vi "EncoderSpeedMise_original.vi"(8 "error in (no error)":errorcluster, 11 "Cluster in":T1={FALSE, "Tick Count(uSec)"=0, "Counter Value"=[0, 0, 0, 0], "x-y"=[0, 0, 0, 0]}) -> (0 "error out":errorcluster, 1 "Updated":bool, 2 "output cluster":T2, 3 "Cluster Out":T1, 4 "Tick Count(uSec)":u32 caption="Tick Count(Ticks)")   [LabVIEW 2018]
uses:
  <vilib>/myRIO/Common/Instrument Driver Framework/myRIO v1.0/Encoder/typedefs/Encoder Signal Mode.ctl
  <vilib>/myRIO/Instrument Drivers/Onboard IO/Encoder/typedefs/Encoder Reference.ctl
  <vilib>/myRIO/Common/Instrument Driver Framework/Utilities/typedefs/myRIO Generic Hardware Reference.ctl
  <vilib>/myRIO/Common/Instrument Driver Framework/Utilities/typedefs/Hardware Version Enum.ctl
  <vilib>/myRIO/Common/Instrument Driver Framework/Utilities/typedefs/myRIO v1.0 Reference.ctl
  <vilib>/myRIO/Common/Instrument Driver Framework/Utilities/typedefs/Generic FPGA Reference.ctl
  <vilib>/myRIO/Common/Instrument Driver Framework/myRIO v1.0/Encoder/typedefs/Encoder Channels Enum.ctl
  <vilib>/myRIO/Common/Instrument Driver Framework/myRIO v1.0/Encoder/typedefs/Encoder Configuration v1.0.ctl
  <vilib>/userdefined/High Color/nirio_resource_hc.ctl
  <vilib>/myRIO/Common/Instrument Driver Framework/Utilities/vis/Is FPGA Ref Available.vi
  <vilib>/myRIO/Common/Instrument Driver Framework/myRIO v1.0/Encoder/vis/myRIO v1.1 Open Encoder.vi
  <vilib>/myRIO/Instrument Drivers/Onboard IO/Encoder/vis/Read.vi
  <vilib>/myRIO/Common/Instrument Driver Framework/Utilities/vis/Validate Channels.vi
  <vilib>/myRIO/Common/Instrument Driver Framework/myRIO v1.0/Encoder/vis/myRIO v1.0 Reserve Encoder.vi
  <vilib>/myRIO/Common/Instrument Driver Framework/myRIO v1.0/Encoder/vis/myRIO v1.0 Build MUX Configuration Encoder.vi
  <vilib>/myRIO/Common/Instrument Driver Framework/myRIO v1.0/Resource Manager/vis/myRIO v1.0 Reserve Channel List.vi
  <vilib>/myRIO/Common/Instrument Driver Framework/myRIO v1.0/Resource Manager/vis/myRIO v1.0 Create Configuration List.vi
  <vilib>/myRIO/Common/Instrument Driver Framework/myRIO v1.0/Resource Manager/vis/myRIO v1.0 Reserve Channel.vi
  <vilib>/myRIO/Common/Instrument Driver Framework/myRIO v1.0/Resource Manager/vis/myRIO v1.0 Unreserve Channel.vi
  <vilib>/myRIO/Common/Instrument Driver Framework/myRIO v1.0/Resource Manager/vis/myRIO v1.0 Build Mutex Name.vi
  <vilib>/Utility/VariantDataType/GetNumericInfo.vi
  <vilib>/Utility/error.llb/Error Cluster From Error Code.vi
  <vilib>/myRIO/Common/Instrument Driver Framework/myRIO v1.0/myRIO v1.1 Open.vi
  <vilib>/myRIO/Common/Instrument Driver Framework/Utilities/vis/IO Manager.vi
  <vilib>/myRIO/Common/Instrument Driver Framework/Utilities/vis/Configuration Manager.vi
  <vilib>/myRIO/Common/Instrument Driver Framework/myRIO v1.0/Resource Manager/vis/myRIO v1.0 Configure IO.vi
  <vilib>/myRIO/Common/Instrument Driver Framework/myRIO v1.0/myRIO v1.0 Close.vi
  <vilib>/myRIO/Common/Instrument Driver Framework/myRIO v1.0/Encoder/vis/myRIO v1.0 Configure Encoder.vi
  <vilib>/myRIO/Common/Instrument Driver Framework/myRIO v1.0/Encoder/vis/myRIO v1.0 Read Encoder.vi
  <vilib>/myRIO/Express VI/Onboard IO/Encoder/Encoder Express VI.xnode
  <vilib>/myRIO/Instrument Drivers/Onboard IO/Encoder/vis/myRIO Encoder Open.xnode
  <vilib>/myRIO/Common/Instrument Driver Framework/myRIO v1.0/Encoder/typedefs/Encoder Count Direction Enum.ctl
  <vilib>/rvi/Arithmetic/AddSubMult/XNode/nirviSatArithmetic.xnode
  <vilib>/myRIO/Instrument Drivers/Onboard IO/Encoder/Encoder.lvlib
panel:
  in  "Reset Encoders":bool
  out "Etu":i32
  out "Taka":i32
  out "Vasen":i32
  out "Oikea":i32
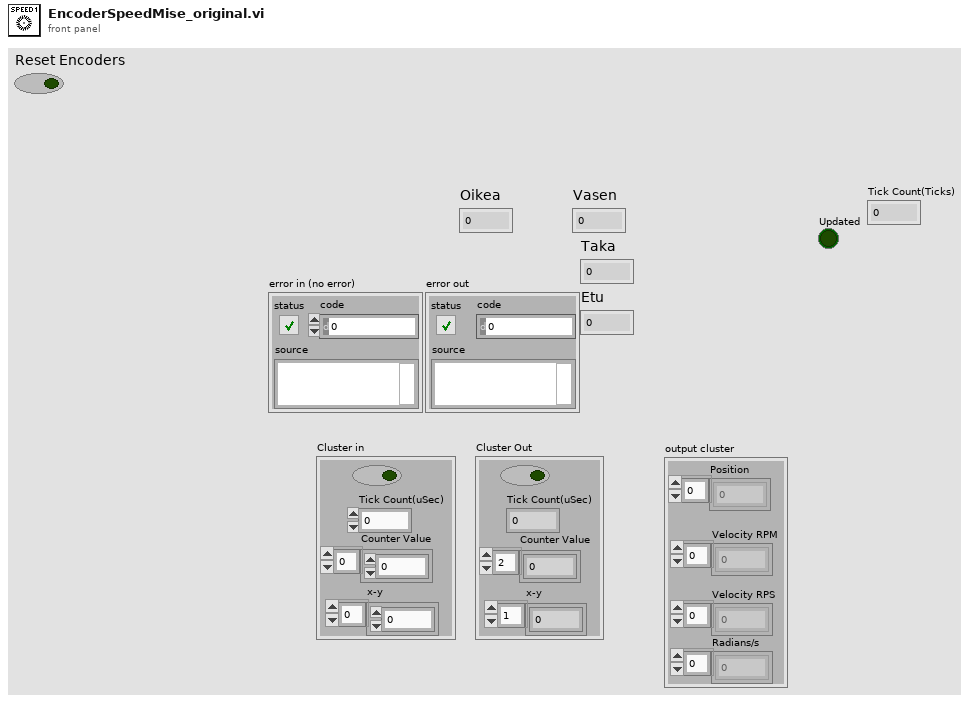
[diagram p1: front panel]
types:
  T1 = cluster{bool, "Tick Count(uSec)":u32, "Counter Value":i32[], "x-y":i32[]}
  T2 = cluster{"Position":i32[], "Velocity RPM":dbl[], "Velocity RPS":dbl[], "Radians/s":dbl[]}
  T3 = cluster{"Counter Value":i32[], dbl[], dbl[], dbl[]}
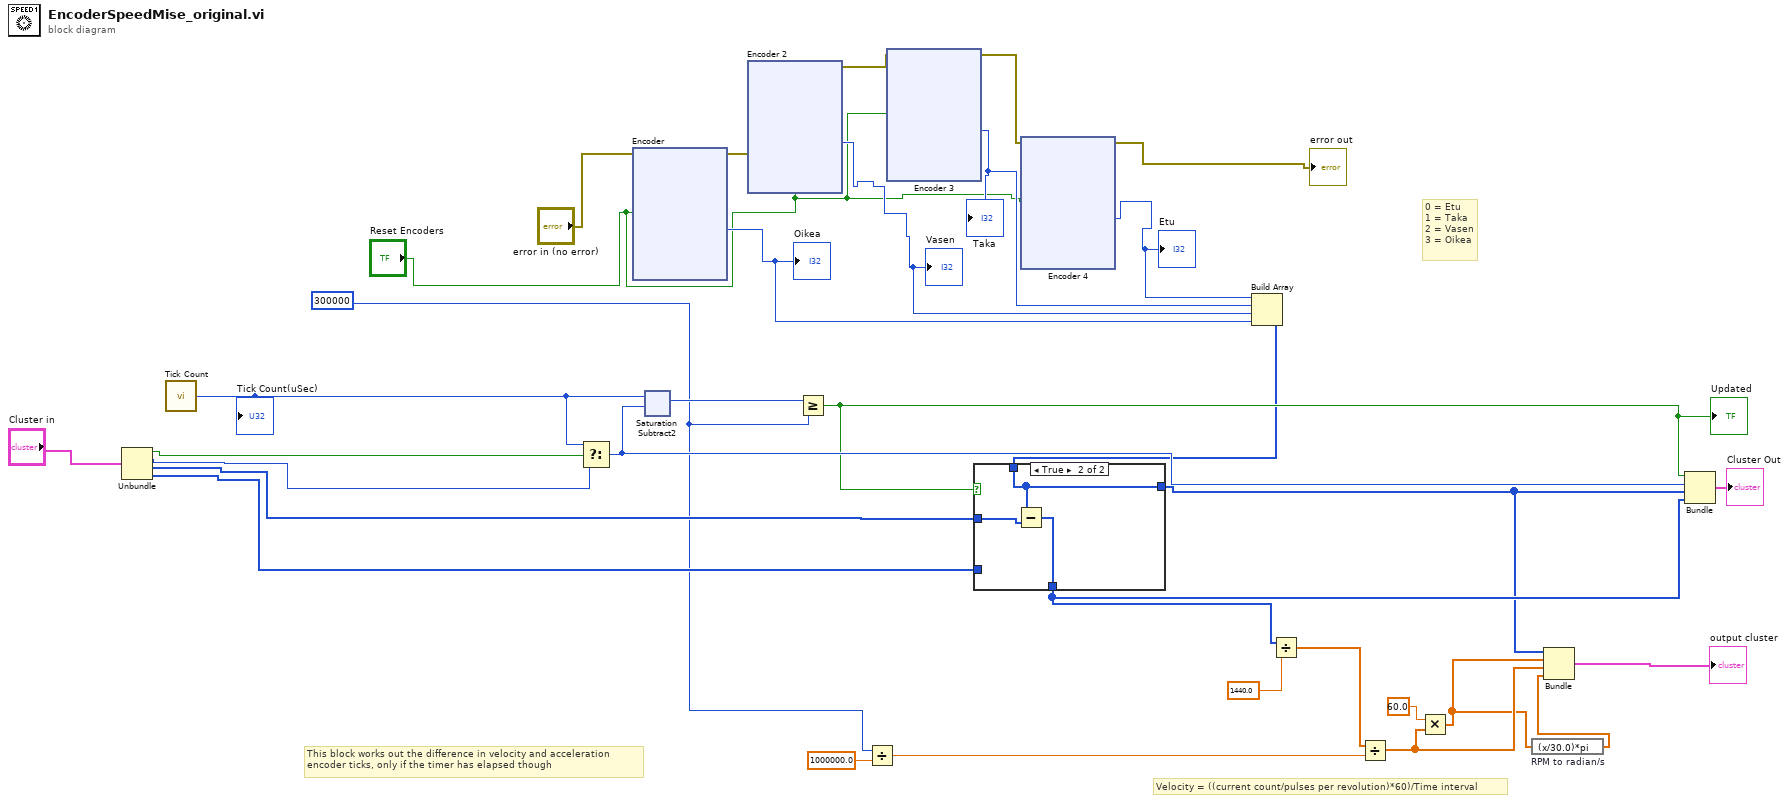
[diagram p0: block diagram]
diagram:
  w2 = 300000
  # "0 = Etu\n1 = Taka\n2 = Vasen\n3 = Oikea"
  # "Velocity = ((current count/pulses per revolution)*60)/Time interval"
  # "This block works out the difference in velocity and acceleration \nencoder ticks, only if the timer has elapsed though"
  n1 = Unbundle("Cluster in") -> (w16:bool, "Tick Count(uSec)"=w15:u32, "Counter Value"=w14:i32[], "x-y"=w13:i32[])
  n2 = call "Tick Count"() -> ("Tick Count(uSec)"=w26:u32)
  "Tick Count(uSec)" <- w26
  n3 = Select(t=w26, s=w16, f=w15) -> (s? t:f=w25:u32)
  n4 = xnode "Encoder"("Reset Counter"="Reset Encoders", "error in (no error)"="error in (no error)") -> ("Counter Value"=w3:i32, "error out"=w20:errorcluster)  [unwired: 2 out]
  "Oikea" <- w3
  n5 = xnode ("Saturation Subtract2")("x"=w26, "y"=w25) -> ("x-y"=w21:u32)
  n6 = xnode "Encoder 2"("Reset Counter"="Reset Encoders", "error in (no error)"=w20) -> ("Counter Value"=w4:i32, "error out"=w9:errorcluster)  [unwired: 2 out]
  "Vasen" <- w4
  n7 = Greater Or Equal?(x=w21, y=w2) -> (x >= y?=w24:bool)
  "Updated" <- w24
  n8 = Divide(x=w2, y=1000000.0) -> (x/y=w28:dbl)
  n9 = xnode "Encoder 3"("Reset Counter"="Reset Encoders", "error in (no error)"=w9) -> ("Counter Value"=w5:i32, "error out"=w8:errorcluster)  [unwired: 2 out]
  "Taka" <- w5
  n10 = xnode "Encoder 4"("Reset Counter"="Reset Encoders", "error in (no error)"=w8) -> ("Counter Value"=w6:i32, "error out"=→"error out":errorcluster)  [unwired: 2 out]
  "Etu" <- w6
  n11 = Build Array(w6, w5, w4, w3) -> (w19:i32[])
  n12 = case shown="True" w24 {
    tunnel: w14 -> [w34 w38]
    tunnel: [w35 w37] -> w29
    tunnel: w13 -> [w35 _]
    tunnel: [w34 w36] -> w27
    tunnel: w19 -> [_ w36]
    frame False {
    }
    frame True {
      n13 = Subtract(x=w36, y=w38) -> (x-y=w37:i32[])
    }
  }
  n14 = Divide(x=w29, y=1440.0) -> (x/y=w30:dbl[])
  n15 = Divide(x=w30, y=w28) -> (x/y=w31:dbl[])
  n16 = Multiply(x=60.0 ("y"), y=w31) -> (x*y=w12:dbl[])
  n17 = expression code="(x/30.0)*pi" "RPM to radian/s"(w12) -> (w11:dbl[])
  n18 = Bundle("Counter Value"=w27, w12, w31, w11) -> (→"output cluster":T3)  [unwired: 1 in]
  n19 = Bundle(w24, "Tick Count(uSec)"=w25, "Counter Value"=w27, "x-y"=w29) -> (→"Cluster Out":T1)  [unwired: 1 in]
